vi "Real Time Run Status.vi"(8 "Error IN":errorcluster) -> (0 "Error OUT":errorcluster, 3 "Real Time Running?":bool caption="*Flashing LED means\nreal-time status is good")   [LabVIEW 2018]
uses:
  <vilib>/NI_Real-Time Target Support.lvlib
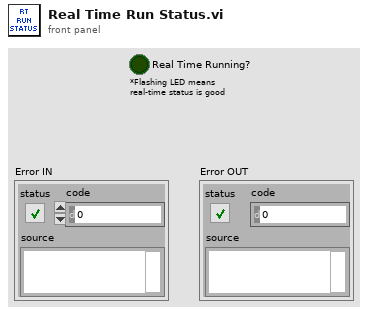
[diagram p1: front panel]
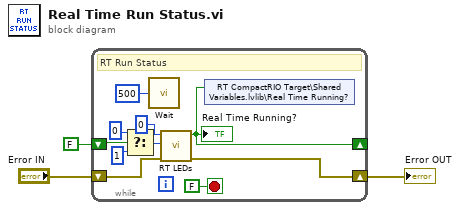
[diagram p0: block diagram]
diagram:
  n1 = while {
    shift-right: [w6] -> _
    shift-left: FALSE -> [w10]
    shift-right: [w4] -> w3
    shift-left: "Error IN" -> [w5]
    stop <- FALSE stop-if-true
    # "RT Run Status"
    n2 = Select(t=0 ("State"), s=w10, f=1 ("State")) -> (s? t:f=w7:i32)
    n3 = call "Wait"("Count(mSec)"=u32 500) -> ()  [unwired: 1 out]
    n4 = call <vilib>:"RT LEDs.vi"("error in (no error)"=w5, "State"=w7, "LED Num"=0 ("State")) -> ("error out"=w4:errorcluster, "Led State"=w6:bool)  [unwired: 3 in]
    "Real Time Running?" <- w6
    n5 = shared-variable "RT CompactRIO Target\\Shared Variables.lvlib\\Real Time Running?"(w6) -> ()  [unwired: 1 in, 1 out]
  }
  "Error OUT" <- w3
